vi "SaveQueueN.vi"(0 "Slider Indexes":cluster{i16, i16, i16}={1, 46, 100}, 1 "Qs and Notis":T14, 2 "Location":enum16{"CUMC", "SERI", "VMR", "Aline", "HSS"}(ring)=enum."Aline", 3 "Append Extra":string, 4 "append letter":i8, 5 "bits A/D":u16=8, 6 "Probe Name":string, 7 "Patient Info":T1={"Eye Selector"=enum."Right", "Plane"=1, "First Name"="", "Last Name"="", "Notes"="", "Patient ID"="", "Scan Location"=enum."Radio Selection 1"} {"Plane" min=1 max=12 step=1 scale=0.0..12.0}, 8 "Scan Info":T13, 10 "Save JPG?":bool, 11 "base path":path, 12 "Motion Settings":T5={"No Motion?"=FALSE, "Motion System"=enum."No Motion Card", "Motion Bd ID"=1, "Motion Profile"="SMAC1", "# Axis"=1, "Reverse Z axis?"=TRUE, "SMAC Axis"=0, "scan pair"=enum."y-(x) scan", "RT fps"=6.0, "Steps per mm"=[1000, 1000, 1000, 1000], "Motor Parameters"={"velocity ct/s"=[10000.0, 10000.0, 10000.0, 50000.0], "accel ct/s^2"=[50000.0, 50000.0, 50000.0, 200000.0]}, "One Way Scan"=FALSE, "Reverse One Way Scan"=FALSE, "Global Position (mm)"=[], "Plane"=0, "Distance between\nscan lines (um)"=0.0, "Distance between\nscan planes (um)"=0.0, "number of scan planes"=1, "Total steps in line"=0, "Xtra plane\ndistance  (um)"=100, "Xtra planes "=1, "Add Axis"=FALSE, "overshoot cts"=200, "BKPT Shift"=0, "Scan Start Time (ms)"=0, "ESP VISA"="GPIB::1::INSTR", "3rd Axis"=1, "GL Ref Out"=refnum, "Galil Address"=""} {"3rd Axis" items=["x", "y", "z", "w"]; "Xtra planes" min=1; "Xtra plane\ndistance  (um)" min=0; "Distance between\nscan planes (um)" format="%.2f"; "Distance between\nscan lines (um)" format="%.2f"; "SMAC Axis" items=["None"=0, "Axis 1"=1, "Axis 2"=2, "Axis 3"=3, "Axis 4"=4, "Axis 5"=5, "Axis 6"=6, "Axis 7"=7, "Axis 8"=8, "Vector Space 1"=17, "Vector Space 2"=18, "Vector Space 3"=19, "Vector Space 4"=20]; "Motion Bd ID" min=1 max=32 step=1}, 13 "Digitizer Settings":T9={"Digitizer delay (us) "=0.0, "rf points per line"=2048, "lines per plane"=128, "Samp Rate (Hz)"=100000000.0, "Additional dig delay (us)"=0.0, "Voltage Scale"=0.4, "Pre-Looks"=0, "Offset delay (us)"=0.0, "bits A/D"=8, "Avg Num"=1, "DigTimeOut"=5.0, "Rel Dig Delay"=0.0, "Dig Ch"=0, "LeCroyCluster"={"LeCroy Channels"=[TRUE, FALSE, FALSE, FALSE], "LC read pt offset"=0.0, "Sweep Avg"=FALSE}, "Main Digitizer"=enum."NI Digitizer", "Dig Config"=enum."Single channel", "Digitizer ID Cluster"={"Acqiris/Alazar/SP ID"=[], "NI Instr Handles"=[], "LeCroy VISA"="", "GaGe Handle"={"Handle"=0, "Sample size"=0, "Resolution"=0, "Offset"=0, "Channels"=0, "Boards"=0}, "ATS Ref"="ATS9350", "Acqiris Address"=["PCI::INSTR0"], "ADQRef"=refnum, "adq_cu_ptr"=refnum}, "Trigger Settings"={"Trig Source"=1, "Trig Coupling"=0, "Trig Slope"=0, "Level (mV)"=1500.0}, "Bulk Acq"=FALSE, "Bulk Start Indexes"=[], "Data Ref RF"=refnum, "NI ID/Channel"=[], "Total Dig CH"=5, "Xtra Ann Trig delay (us)"=10.0, "Fix Z Delay?"=FALSE, "One Way Transmission?"=FALSE, "Data Ref Log"=refnum} {"Trigger Settings"."Trig Slope" items=["Positive", "Negative"]; "Trigger Settings"."Level (mV)" format="%.2f"; "Trigger Settings"."Trig Coupling" items=["DC 1 MOhm", "AC 1 MOhm", "DC 50 Ohm", "AC 50 Ohm"]; "Trigger Settings"."Trig Source" items=["Chan 1", "External"]; "Rel Dig Delay" format="%.2f"; "DigTimeOut" format="%.2f"; "Avg Num" min=1; "Offset delay (us)" format="%.2f"; "Additional dig delay (us)" format="%.2f"; "Digitizer delay (us)" format="%.2f"}, 19 "Ann Array Params":T2={"Synth Foc?"=FALSE, "Focal Zones"=41, "Switch T/R"=0, "Trans Geometry (mm)"={"Transducer"=0, "Geo Focus"=12.0, "a (radius)"=3.0, "# of rings"=5, "kerf space "=0.1, "Center Freq"=12.0}, "Sub Ap Excite?"=FALSE, "Full Array Scan?"=FALSE, "Xmt/Rcv"={"XMIT"=[TRUE, TRUE, TRUE, TRUE, TRUE], "RCV"=[TRUE, TRUE, TRUE, TRUE, TRUE]}, "PulseSpacing (us)"=0.0, "Xmit Ring"=0, "XMIT CHS"=0, "RCV CHS"=0, "GPU?"=FALSE, "Save TIFF?"=FALSE, "downfactor"=1, "RCV 1CH"=0} {"RCV 1CH" items=["All", "1", "2", "3", "4", "5"]; "Trans Geometry (mm)"."Transducer" items=["6D 12R 40 MHz"=0, "10D 31R 20 MHz"=1, "10D 23R 20 MHz"=2, "6D 23R 40 MHz"=3, "4.5D 10.7R 40 MHz"=4, "9D 23.5R 20 MHz"=5, "9D 25.8R 20MHz"=6, "Enter"=99]; "Switch T/R" min=1 max=5 step=1}) -> (14 "append letter out":i8)   [LabVIEW 2022 SP3]
uses:
  <vilib>/picture/picture.llb/imagedata.ctl
  ScanningControl/Digitizers/-DigitizerRoutines/DigitizerSettings.ctl
  ScanningControl/Digitizers/-DigitizerRoutines/Digitizer.ctl
  ScanningControl/Digitizers/-DigitizerRoutines/DigConfig.ctl
  ScanningControl/Digitizers/-DigitizerRoutines/DigitizerID.ctl
  C:/Windows/System32/ADQAPI_dotNet_helper.dll
  Windows/System32/ADQAPI_dotNet_helper.dll
  ScanningControl/Motion Controllers/NI_controller/-NI_MotionRoutines/MotionParameters.ctl
  ScanningControl/Motion Controllers/NI_controller/-NI_MotionRoutines/MotionSys.ctl
  ScanningControl/Motion Controllers/-MotionRoutines/ScanAxis.ctl
  ScanningControl/Motion Controllers/-MotionRoutines/3rdAxis.ctl
  Annular Array/-AnnularRoutines/AnnularArray.ctl
  Annular Array/-AnnularRoutines/TransGeometry.ctl
  Annular Array/-AnnularRoutines/ArrayGeometry.ctl
  PatientInfoDef.ctl
panel:
  # "1-D and 2-D B scan settings"
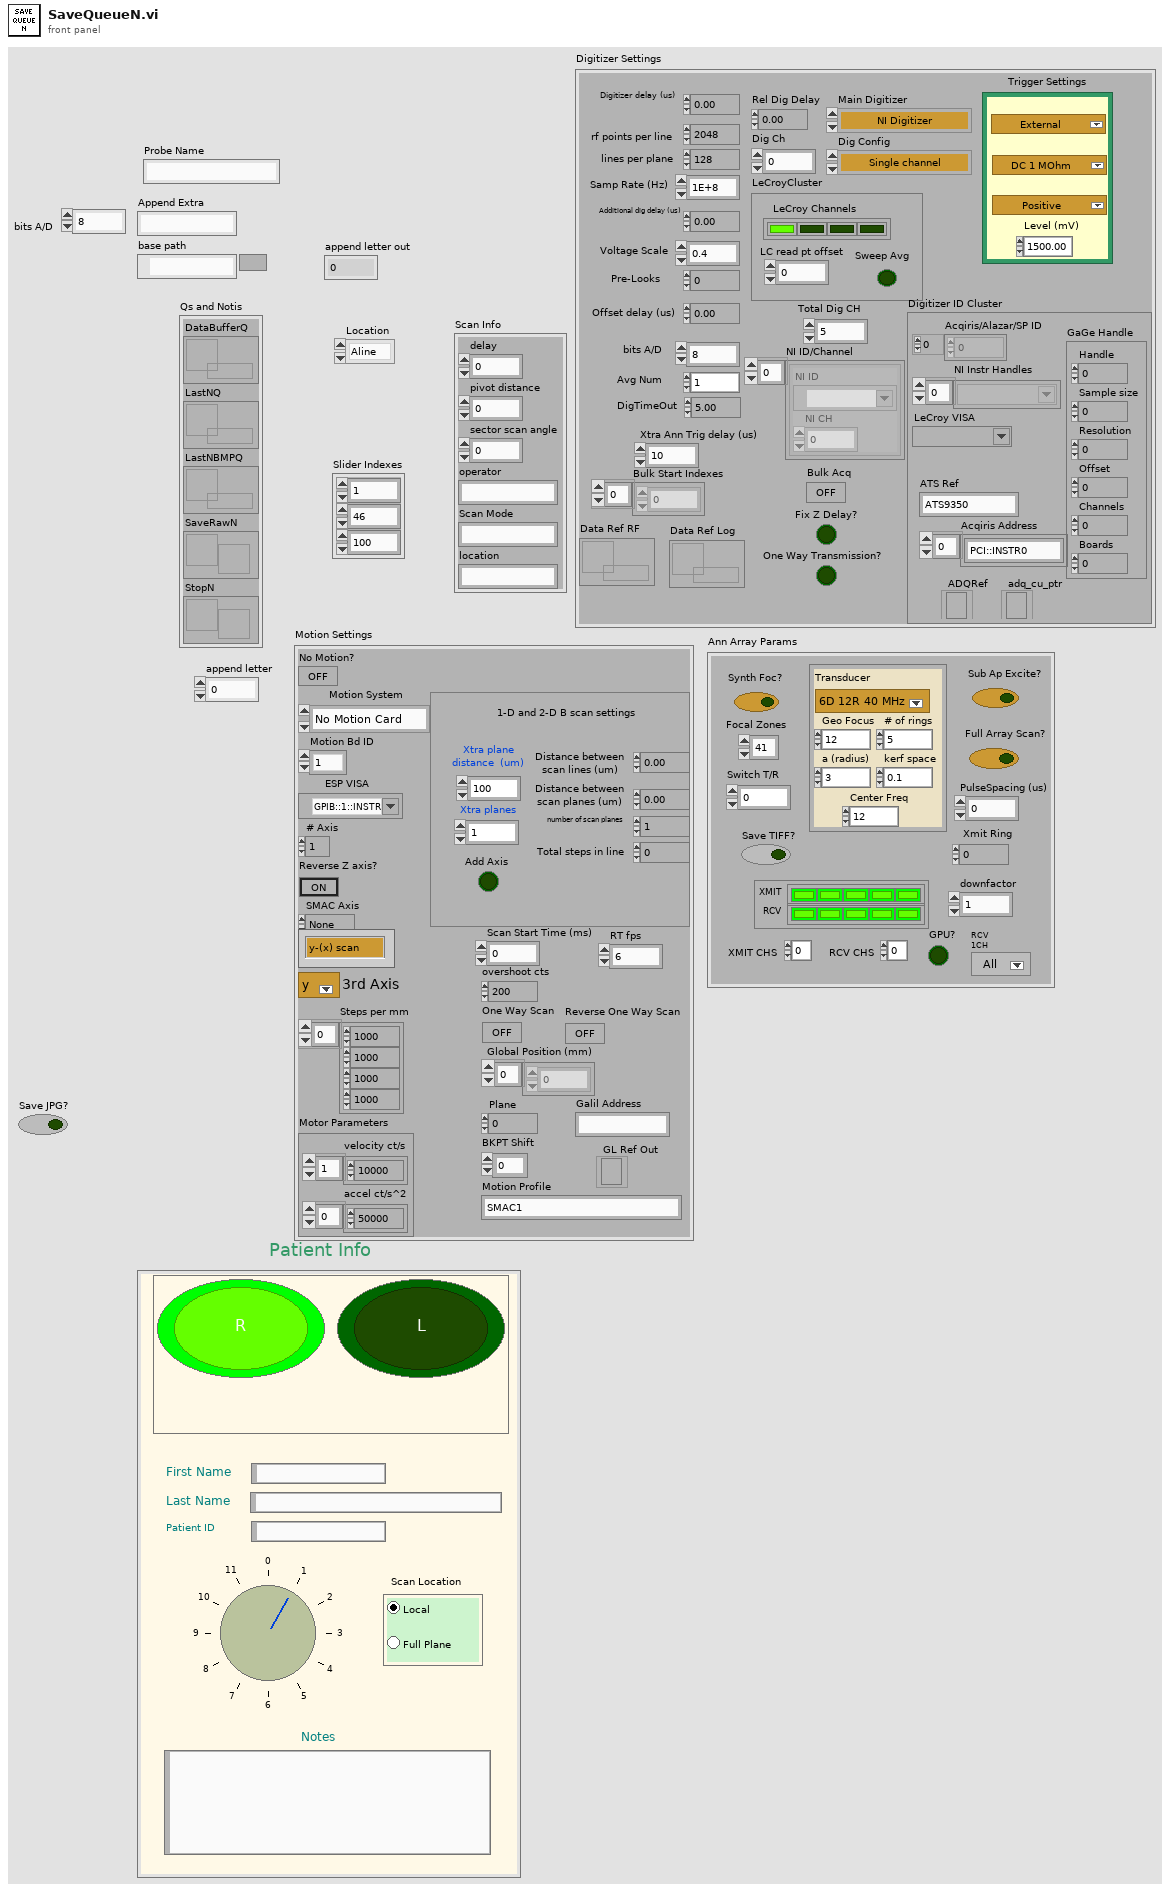
[diagram p1: front panel]
types:
  T1 = typedef "PatientInfoDef.ctl" = cluster{"Eye Selector":enum32{"Left", "Right"}, "Plane":i8, "First Name":string, "Last Name":string, "Notes":string, "Patient ID":string, "Scan Location":enum32{"Radio Selection 1", "Radio Selection 2"}}
  T2 = typedef "AnnularArray.ctl" = cluster{"Synth Foc?":bool, "Focal Zones":i16, "Switch T/R":i16, "Trans Geometry (mm)":T3, "Sub Ap Excite?":bool, "Full Array Scan?":bool, "Xmt/Rcv":cluster{"XMIT":bool[], "RCV":bool[]}, "PulseSpacing (us)":sgl, "Xmit Ring":i32, "XMIT CHS":u8, "RCV CHS":u8, "GPU?":bool, "Save TIFF?":bool, "downfactor":i32, "RCV 1CH":u16}
  T3 = typedef "TransGeometry.ctl" = cluster{"Transducer":T4, "Geo Focus":dbl, "a (radius)":dbl, "# of rings":i32, "kerf space ":dbl, "Center Freq":dbl}
  T4 = typedef "ArrayGeometry.ctl" = u16
  T5 = typedef "MotionParameters.ctl" = cluster{"No Motion?":bool, "Motion System":T6, "Motion Bd ID":u8, "Motion Profile":string, "# Axis":i8, "Reverse Z axis?":bool, "SMAC Axis":u16, "scan pair":T7, "RT fps":sgl, "Steps per mm":i32[], "Motor Parameters":cluster{"velocity ct/s":dbl[], "accel ct/s^2":dbl[]}, "One Way Scan":bool, "Reverse One Way Scan":bool, "Global Position (mm)":dbl[], "Plane":i32, "Distance between\nscan lines (um)":sgl, "Distance between\nscan planes (um)":sgl, "number of scan planes":i32, "Total steps in line":i32, "Xtra plane\ndistance  (um)":i32, "Xtra planes ":i32, "Add Axis":bool, "overshoot cts":i32, "BKPT Shift":i32, "Scan Start Time (ms)":u32, "ESP VISA":refnum<visa-resource-name>, "3rd Axis":T8, "GL Ref Out":refnum<k7>, "Galil Address":string}
  T6 = typedef "MotionSys.ctl" = enum16{"MM3000", "NI 735x", "Newport ESP", "No Motion Card", "Galil"}
  T7 = typedef "ScanAxis.ctl" = enum16{"y-(x) scan", "x-(y) scan", "z-(x) scan", "z-(y) scan", "y-(z) scan", "x-(z) scan", "w-(x) scan", "w-(y) scan", "w-(z) scan", "x-(w) scan", "y-(w) scan", "z-(w) scan"}
  T8 = typedef "3rdAxis.ctl" = u16
  T9 = typedef "DigitizerSettings.ctl" = cluster{"Digitizer delay (us) ":dbl, "rf points per line":i32, "lines per plane":i32, "Samp Rate (Hz)":dbl, "Additional dig delay (us)":dbl, "Voltage Scale":dbl, "Pre-Looks":i32, "Offset delay (us)":dbl, "bits A/D":i8, "Avg Num":i32, "DigTimeOut":sgl, "Rel Dig Delay":sgl, "Dig Ch":i32, "LeCroyCluster":cluster{"LeCroy Channels":bool[], "LC read pt offset":dbl, "Sweep Avg":bool}, "Main Digitizer":T10, "Dig Config":T11, "Digitizer ID Cluster":T12, "Trigger Settings":cluster{"Trig Source":u16, "Trig Coupling":u16, "Trig Slope":u16, "Level (mV)":dbl}, "Bulk Acq":bool, "Bulk Start Indexes":i32[], "Data Ref RF":refnum<data-value>, "NI ID/Channel":cluster{"NI ID":refnum<k15>, "NI CH":i32}[], "Total Dig CH":i32, "Xtra Ann Trig delay (us)":dbl, "Fix Z Delay?":bool, "One Way Transmission?":bool, "Data Ref Log":refnum<data-value>}
  T10 = typedef "Digitizer.ctl" = enum16{"Acqiris Digitizer", "NI Digitizer", "LeCroy", "GaGe", "AlazarTech", "No Digitizer", "Teledyne"}
  T11 = typedef "DigConfig.ctl" = enum16{"Single channel", "2 Chans w/ 2 Acqiris", "2 Chans w/ 1 Acqiris", "5-CH Pulser New", "5-CH pulser w/ ann array", "5-pass style ann array", "Empty"}
  T12 = typedef "DigitizerID.ctl" = cluster{"Acqiris/Alazar/SP ID":u32[], "NI Instr Handles":refnum<k15>[], "LeCroy VISA":refnum<visa-resource-name>, "GaGe Handle":cluster{"Handle":u32, "Sample size":u32, "Resolution":i32, "Offset":i32, "Channels":u32, "Boards":u32}, "ATS Ref":string, "Acqiris Address":string[], "ADQRef":refnum<k24>, "adq_cu_ptr":refnum<k24>}
  T13 = cluster{"delay":sgl, "pivot distance":sgl, "sector scan angle":sgl, "operator":string, "Scan Mode":string, "location":string}
  T14 = cluster{"DataBufferQ":refnum<queue>, "LastNQ":refnum<queue>, "LastNBMPQ":refnum<queue>, "SaveRawN":refnum<notifier>, "StopN":refnum<notifier>}
  T15 = typedef "imagedata.ctl" = cluster{"image type":i32, "image depth":i32, "image":u8[], "mask":u8[], "colors":u32[], "Rectangle":cluster{"left":i16, "top":i16, "right":i16, "bottom":i16}}
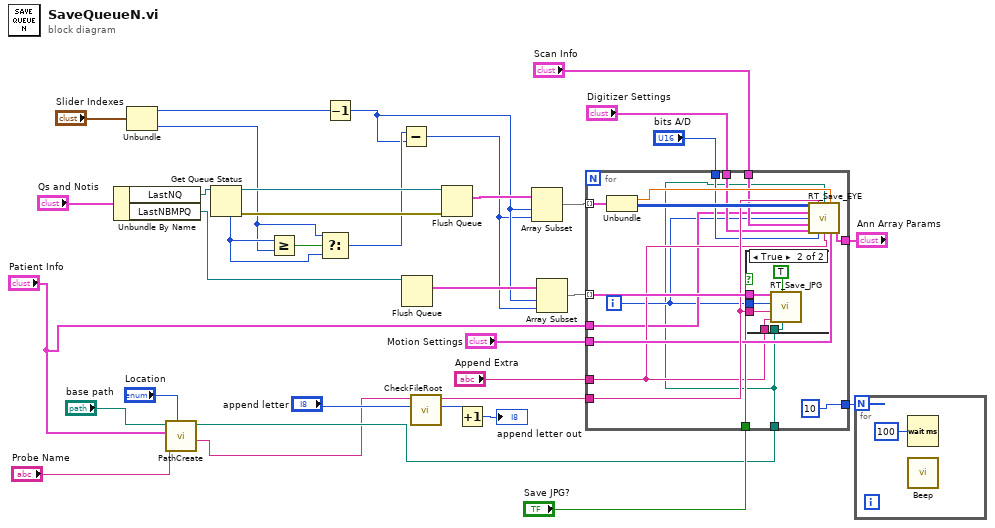
[diagram p0: block diagram]
diagram:
  n1 = Unbundle By Name("Qs and Notis") -> ("LastNQ"=w18:refnum<queue>, "LastNBMPQ"=w19:refnum<queue>)
  n2 = Unbundle("Slider Indexes") -> (w23:i16, w25:i16)  [unwired: 1 out]
  n3 = call "PathCreate.vi"("Location"="Location", "Probe Name"="Probe Name", "Patient Info"="Patient Info", "base path"="base path") -> ("FileName"=w3:string, "appended path"=w4:path)  [unwired: 6 in]
  n4 = Get Queue Status(queue=w18) -> (queue out=w31:refnum<queue>, error out=w32:errorcluster, # elements in queue=w35:i32)  [unwired: 2 in, 5 out]
  n5 = Greater Or Equal?(x=w35, y=w25) -> (x >= y?=w34:bool)
  n6 = Select(t=w25, s=w34, f=w35) -> (s? t:f=w24:i32)
  n7 = Decrement(x=w23) -> (x-1=w22:i16)
  n8 = Subtract(x=w24, y=w22) -> (x-y=w21:i32)
  n9 = Flush Queue(queue=w19) -> (remaining elements=w27:T15[])  [unwired: 1 in, 2 out]
  n10 = call "CheckFileRoot.vi"("append letter"="append letter", "File Name"=w3) -> ("append letter out"=w13:i8, "FileNameOut"=w14:string)  [unwired: 8 in]
  n11 = Flush Queue(queue=w31, error in (no error)=w32) -> (remaining elements=w29:cluster{"gain":dbl, "wfm":i16[][]}[])  [unwired: 2 out]
  n12 = Increment(x=w13) -> (x+1=→"append letter out":i8)
  n13 = Array Subset(array=w29, index=w22, length=w21) -> (w28:cluster{"gain":dbl, "wfm":i16[][]}[])
  n14 = Array Subset(array=w27, index=w22, length=w21) -> (w26:T15[])
  n15 = for {
    tunnel: w28 -> [w49] mode=indexing
    tunnel: w14 -> [w47]
    tunnel: w26 -> [w48] mode=indexing
    tunnel: "Scan Info" -> [w46]
    tunnel: "bits A/D" -> [w45]
    tunnel: [10] -> w15
    tunnel: "Digitizer Settings" -> [w43]
    tunnel: "Motion Settings" -> [w42]
    tunnel: "Ann Array Params" -> [w41]
    tunnel: "Save JPG?" -> [w40]
    tunnel: "Append Extra" -> [w39]
    tunnel: "Patient Info" -> [w38]
    tunnel: w4 -> [w36]
    i -> [w37]
    n16 = Unbundle(w49) -> ("gain"=w51:dbl, "wfm"=w50:i16[][])
    n17 = case shown="True" w40 {
      tunnel: w48 -> [_ w57]
      tunnel: w47 -> [_ w56]
      tunnel: w37 -> [_ w55]
      tunnel: w39 -> [_ w53]
      tunnel: w36 -> [_ w52]
      frame False {
      }
      frame True {
        n18 = call "RT_Save_JPG.vi"("base path"=w52, "BMP(T)/JPG(F)"=TRUE, "Append Extra"=w53, "Movie Name"=w56, "Frame"=w55, "image data"=w57) -> ()  [unwired: 6 in]
      }
    }
    n19 = call "RT_Save_EYE.vi"("Data"=w50, "Eye Name"=w47, "Save Directory"=w36, "Digitizer Gain"=w51, "Patient Info"=w38, "Frame"=w37, "Scan Info"=w46, "Digitizer Settings"=w43, "bits A/D"=w45, "File Append"=w39, "Motion Settings"=w42, "Ann Array Params"=w41) -> ()  [unwired: 4 in]
  }
  n20 = for {
    N: w15 -> [_]
    n21 = Wait (ms)(milliseconds to wait=u32 100) -> ()  [unwired: 1 out]
    n22 = call <vilib>:"Beep.vi"() -> ()  [unwired: 12 in]
  }
